vi "Result Update.vi"(7 "MultiList Ref":refnum<vi>, 8 "error in (no error)":errorcluster, 9 "Real Coordinates":cluster{"X":dbl, "Y":dbl}[](array[cluster])=[{"X"=330.0, "Y"=330.0}, {"X"=340.0, "Y"=330.0}, {"X"=330.0, "Y"=340.0}], 10 "Pixel Coordinates":cluster{"X":dbl, "Y":dbl}[](array[cluster])=[{"X"=330.0, "Y"=330.0}, {"X"=340.0, "Y"=330.0}, {"X"=330.0, "Y"=340.0}]) -> (0 "error out":errorcluster)   [LabVIEW 2015]
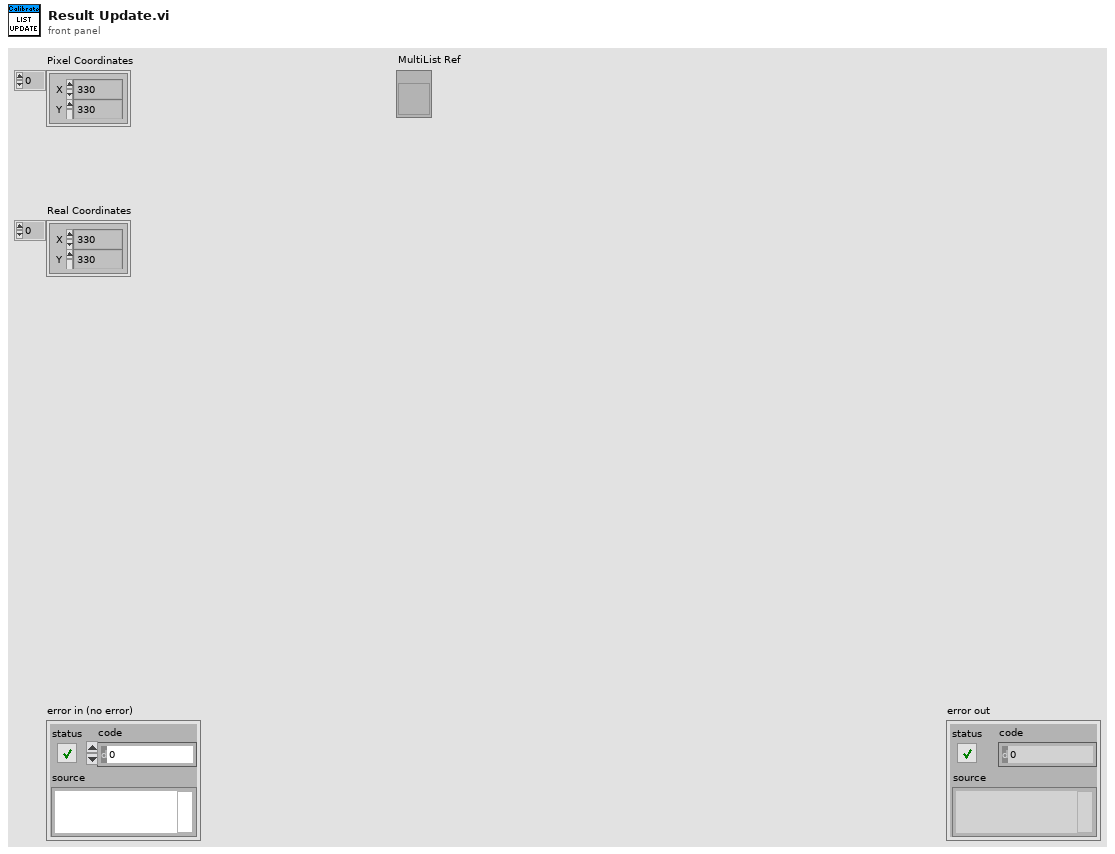
[diagram p1: front panel]
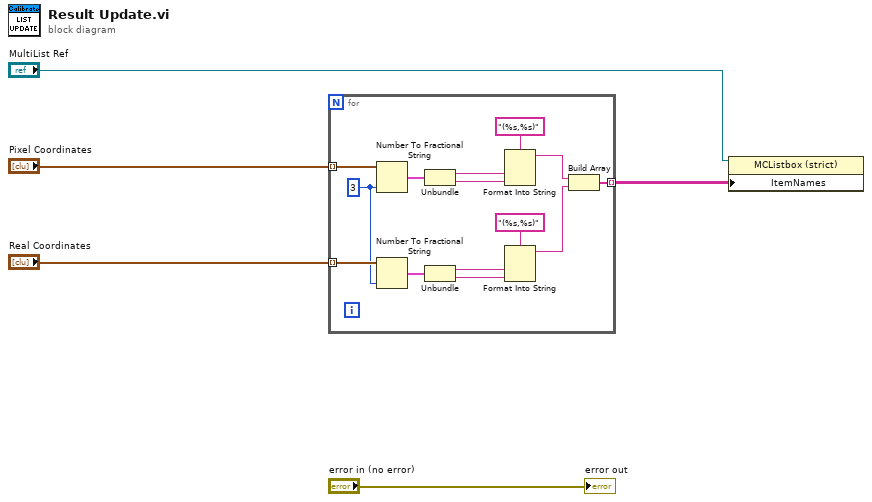
[diagram p0: block diagram]
diagram:
  n1 = for {
    tunnel: "Pixel Coordinates" -> [w19] mode=indexing
    tunnel: "Real Coordinates" -> [w18] mode=indexing
    tunnel: [w8] -> w2 mode=indexing
    w7 = i16 3 ("precision (6)")
    n2 = Number To Fractional String(number=w19, precision (6)=w7) -> (F-format string=w17:cluster{"X":string, "Y":string})  [unwired: 2 in]
    n3 = Number To Fractional String(number=w18, precision (6)=w7) -> (F-format string=w10:cluster{"X":string, "Y":string})  [unwired: 2 in]
    n4 = Unbundle(w17) -> ("X"=w16:string, "Y"=w15:string)
    n5 = Unbundle(w10) -> ("X"=w11:string, "Y"=w12:string)
    n6 = Format Into String(format string="(%s,%s)", w16, w15) -> (resulting string=w6:string)  [unwired: 2 in, 1 out]
    n7 = Format Into String(format string="(%s,%s)", w11, w12) -> (resulting string=w9:string)  [unwired: 2 in, 1 out]
    n8 = Build Array(w6, w9) -> (w8:string[])
  }
  n9 = property class="MCListbox (strict)"(reference="MultiList Ref", "ItemNames"=w2) -> ()  [unwired: 1 in, 2 out]
  "error out" <- "error in (no error)"
